vi "Measure ALL in 3Phase State.vi"(8 "error in":errorcluster, 10 "Phase":enum16{"A", "B", "C"}(ring), 11 "VISA resource name":refnum<visa-resource-name>) -> (0 "error out":errorcluster, 2 "Measurement":string, 3 "VISA resource name out":refnum<visa-resource-name>)   [LabVIEW 2015, in "IT-M7700.lvlib"]
doc: "This command is used to reread Vrms, Vdc, Irms, Idc, Ipk_plus, Ipk_minus, W (Real Power), PF, IPmax, VA, Q (VAR), VTHD, Freq, Vpeak, VAC, IAC, ITHD17 set of values."
uses:
  <instrlib>/IT-M7700/IT-M7700.lvlib
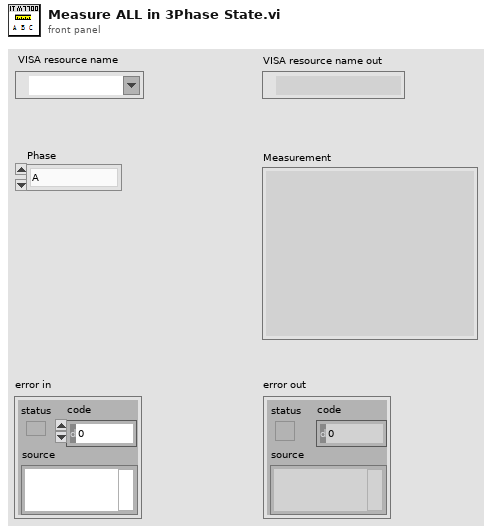
[diagram p1: front panel]
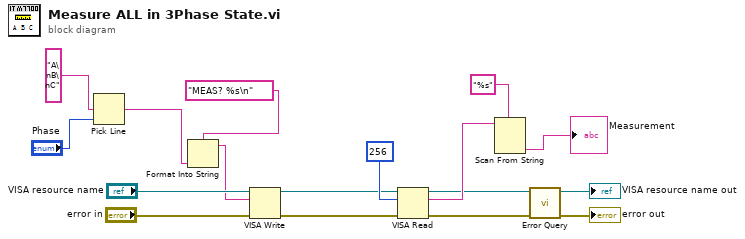
[diagram p0: block diagram]
diagram:
  n1 = Pick Line(multi-line string="A\nB\nC" ("多行字符串"), line index="Phase") -> (output string=w2:string)  [unwired: 1 in]
  n2 = Format Into String(format string="MEAS? %s\n", w2) -> (resulting string=w1:string)  [unwired: 2 in, 1 out]
  n3 = VISA Write(VISA resource name="VISA resource name", write buffer=w1, error in (no error)="error in") -> (VISA resource name out=w7:refnum<visa-resource-name>, error out=w6:errorcluster)  [unwired: 1 out]
  n4 = VISA Read(VISA resource name=w7, byte count=256, error in (no error)=w6) -> (VISA resource name out=w12:refnum<visa-resource-name>, read buffer=w17:string, error out=w8:errorcluster)  [unwired: 1 out]
  n5 = Scan From String(format string="%s", input string=w17) -> (output 1=→"Measurement":string)  [unwired: 3 in, 3 out]
  n6 = call <instrlib>:"Error Query.vi"("error in"=w8, "VISA resource name"=w12) -> ("error out"=→"error out":errorcluster, "VISA resource name out"=→"VISA resource name out":refnum<visa-resource-name>)  [unwired: 6 in, 2 out]
